vi "Destroy Events.vi"(8 "error in (no error)":errorcluster, 11 "Log_Engine in":refnum<class "Log_Engine.lvclass">) -> (0 "error out":errorcluster, 3 "Log_Engine out":refnum<class "Log_Engine.lvclass">)   [LabVIEW 2019, in "Log_Engine.lvclass"]
doc: "Developed by Kevin Thompson\nkevin@thompsonengineering.net\n\nCopyright 2018\nThompson Engineering, LLC"
uses:
  Log_Engine.lvclass
  Log_Engine.lvclass/Log_Engine.ctl
  Accessors/Get PublicEvents.vi
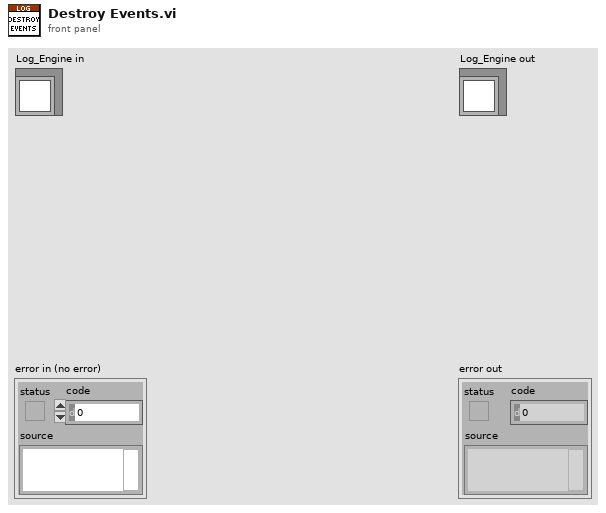
[diagram p1: front panel]
types:
  T1 = typedef "Log_Engine.lvclass/Public Events--cluster.ctl" = cluster{"Log_Engine.AsyncCmd Event":refnum<user-event>, "Log_Engine.AsyncMsg Event":refnum<user-event>, "stop process":refnum<user-event>, "Log_Engine.LogStateChg Ev":refnum<user-event>, "Log_Engine.TDMSStateChg Ev":refnum<user-event>}
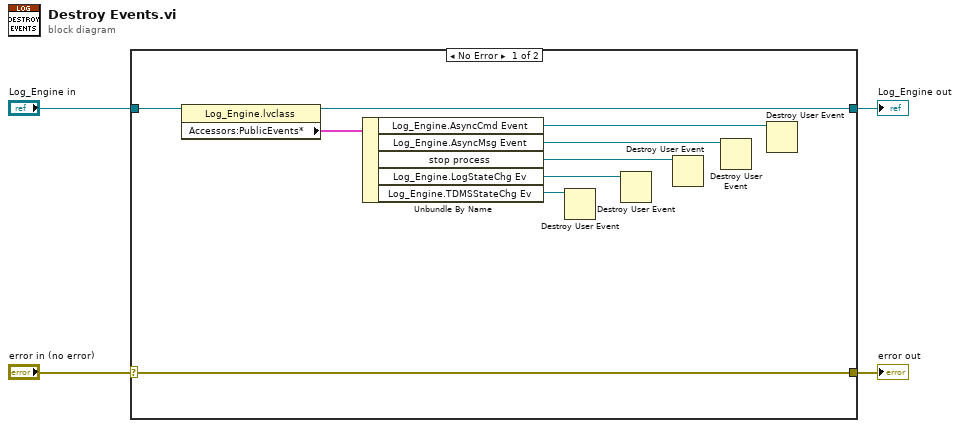
[diagram p0: block diagram]
diagram:
  n1 = case shown="No Error" "error in (no error)" {
    selector: "error in (no error)" -> [w9 w15]
    tunnel: [w9 w15] -> w3
    tunnel: [w12 w14] -> w1
    tunnel: "Log_Engine in" -> [w13 w14]
    frame No Error {
      n2 = property class="Log_Engine.lvclass"(reference=w13) -> (reference out=w12:refnum<class "Log_Engine.lvclass">, "Accessors:PublicEvents*"=w11:T1)  [unwired: 1 in, 1 out]
      n3 = Unbundle By Name(w11) -> ("Log_Engine.AsyncCmd Event"=w10:refnum<user-event>, "Log_Engine.AsyncMsg Event"=w8:refnum<user-event>, "stop process"=w7:refnum<user-event>, "Log_Engine.LogStateChg Ev"=w5:refnum<user-event>, "Log_Engine.TDMSStateChg Ev"=w6:refnum<user-event>)
      n4 = Destroy User Event(user event=w6) -> ()  [unwired: 1 in, 1 out]
      n5 = Destroy User Event(user event=w5) -> ()  [unwired: 1 in, 1 out]
      n6 = Destroy User Event(user event=w7) -> ()  [unwired: 1 in, 1 out]
      n7 = Destroy User Event(user event=w8) -> ()  [unwired: 1 in, 1 out]
      n8 = Destroy User Event(user event=w10) -> ()  [unwired: 1 in, 1 out]
    }
    frame Error {
    }
  }
  "error out" <- w3
  "Log_Engine out" <- w1
